vi "PreUninstall.RemoveFiles.vi"(8 "error in (no error)":errorcluster, 11 "TestStand Components\\TypePalettes Directory":path) -> (0 "error out":errorcluster)   [LabVIEW 2013]
uses:
  Types/Components Directory Install Files String Array.ctl
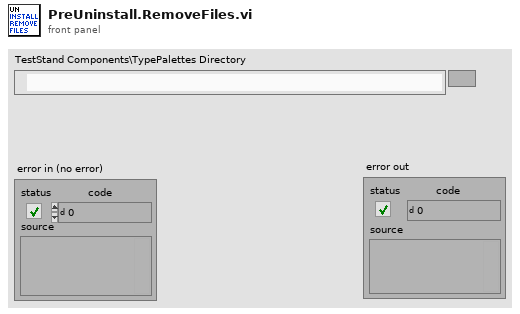
[diagram p1: front panel]
types:
  T1 = typedef "Components Directory Install Files String Array.ctl" = string[]
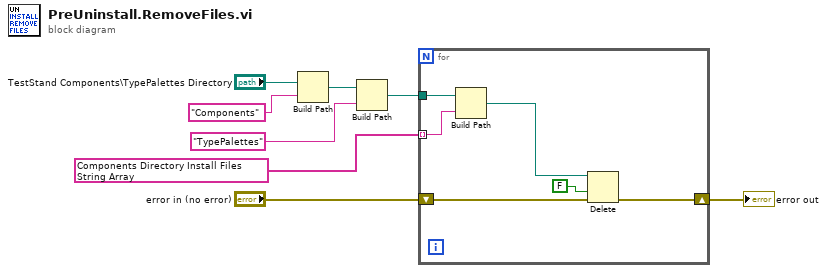
[diagram p0: block diagram]
diagram:
  n1 = Build Path(base path="TestStand Components\\TypePalettes Directory", name or relative path="Components") -> (appended path=w3:path)
  n2 = Build Path(base path=w3, name or relative path="TypePalettes") -> (appended path=w1:path)
  n3 = for {
    tunnel: T1 ["MiscHelperVIs.lvlibp", "RTSequenceVIs.lvlibp", "Set Channels.lvlibp", "Logging.lvlibp", "NI_VeristandTypes.ini", "Veristand_icon_vista.ico"] ("Array") -> [w14] mode=indexing
    shift-right: [w10] -> w6
    shift-left: "error in (no error)" -> [w11]
    tunnel: w1 -> [w9]
    n4 = Build Path(base path=w9, name or relative path=w14) -> (appended path=w13:path)
    n5 = Delete(path (use dialog)=w13, confirm (F)=FALSE, error in=w11) -> (error out=w10:errorcluster)  [unwired: 2 in, 2 out]
  }
  "error out" <- w6
